vi "Test Arduino-Adafruit stepper API.vi"() -> ()   [LabVIEW 2020]
doc: "Arduino-Adafruit stepper API Tester."
uses:
  Arduino stepper library/Public/Controls/Com Port Options.ctl
  Arduino stepper library/Public/Controls/Motor initialization parameters--cluster.ctl
  Arduino stepper library/Public/Controls/Motor direction.ctl
  Arduino stepper library/Public/Controls/Move motor parameters--cluster.ctl
  Arduino stepper library/Public/Controls/Step style.ctl
  <vilib>/Utility/error.llb/DialogType.ctl
  Arduino-Adafruit stepper.lvlib
  Arduino stepper library/Control de MaP.lvlib
panel:
  in  "Stop movement":bool
  in  "Timeout":i32=50
  in  "Move parameters":T1={"Action"=1, "Direction motor 1"=1, "Direction motor 2"=1, "Steps motor 1"=200, "Steps motor 2"=200, "Step style motor 1"=1, "Step style motor 2"=1} {"Step style motor 2" items=["", "Single", "Double", "Interleave", "Microstep"]; "Step style motor 1" items=["", "Single", "Double", "Interleave", "Microstep"]; "Direction motor 2" items=["", "Forward", "Backward"]; "Direction motor 1" items=["", "Forward", "Backward"]; "Action" items=["", "Initialize", "Move"]}
  in  "Begin movement":bool
  in  "Home direction (M2)":T2=1 items=["", "Forward", "Backward"]
  in  "Home direction (M1)":T2=1 items=["", "Forward", "Backward"]
  in  "Home motors":bool
  out "Motors ready?":bool
  in  "Comando":T4={"Action"=0, "Steps per rev motor 1"=200, "Steps per rev motor 2"=200, "RPM motor 1"=400, "RPM motor 2"=400} {"Action" items=["Initialize", "Move"]}
  in  "Init motors":bool
  out "Connected?":bool
  in  "Disconnect":bool
  in  "COM options":T5={"baud rate"=115200, "data bits"=8, "parity"=enum."None"} {"data bits" min=5 max=8 step=1}
  in  "VISA resource name":refnum<visa-resource-name>
  in  "Connect":bool
  out "last error":errorcluster
  in  "Show Diagram on Init":bool
  in  "Run as Singleton?":bool
  in  "Show Block Diagram":bool
  in  "Refresh Modules":bool
  out "Active Modules":string[](array[string])
  in  "Stop Module":bool
  in  "Select Module":i32(ring)=-1 caption="Select Module\nTo send Request to" items=["All"=-1]
  in  "Run New Module":bool
  in  "Hide Module Panel":bool
  in  "Show Module Panel":bool
  out "Status":string
  # "This VI tests the API for the Module."
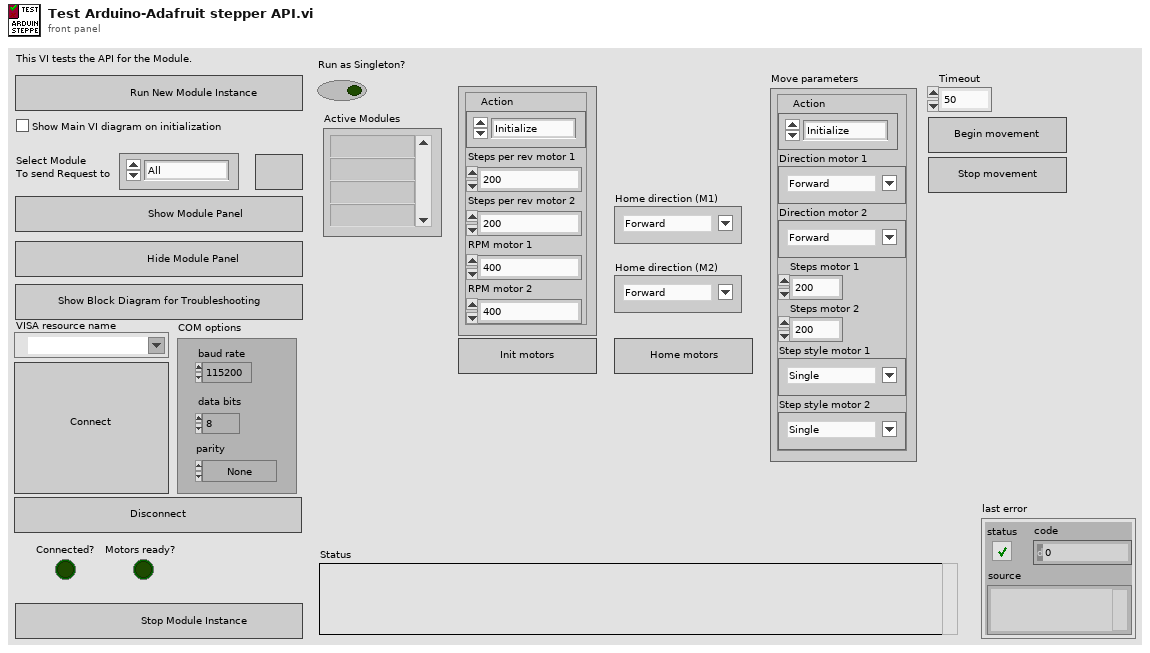
[diagram p1: front panel]
types:
  T1 = typedef "Control de MaP.lvlib/Move motor parameters--cluster.ctl" = cluster{"Action":u8, "Direction motor 1":T2, "Direction motor 2":T2, "Steps motor 1":u16, "Steps motor 2":u16, "Step style motor 1":T3, "Step style motor 2":T3}
  T2 = typedef "Control de MaP.lvlib/Motor direction.ctl" = u8
  T3 = typedef "Control de MaP.lvlib/Step style.ctl" = u8
  T4 = typedef "Control de MaP.lvlib/Motor initialization parameters--cluster.ctl" = cluster{"Action":u8, "Steps per rev motor 1":u8, "Steps per rev motor 2":u8, "RPM motor 1":u16, "RPM motor 2":u16}
  T5 = typedef "Control de MaP.lvlib/Com Port Options.ctl" = cluster{"baud rate":u32, "data bits":u16, "parity":enum16{"None", "Odd", "Even", "Mark", "Space"}}
  T6 = typedef "Arduino-Adafruit stepper.lvlib/Broadcast Events--cluster.ctl" = cluster{"Module Did Init":refnum<user-event>, "Status Updated":refnum<user-event>, "Error Reported":refnum<user-event>, "Module Did Stop":refnum<user-event>, "Update Module Execution Status":refnum<user-event>, "Connection successful":refnum<user-event>, "Connection failed":refnum<user-event>, "Device disconnected":refnum<user-event>, "Motors ready":refnum<user-event>, "System busy":refnum<user-event>}
  T7 = typedef "DialogType.ctl" = u16
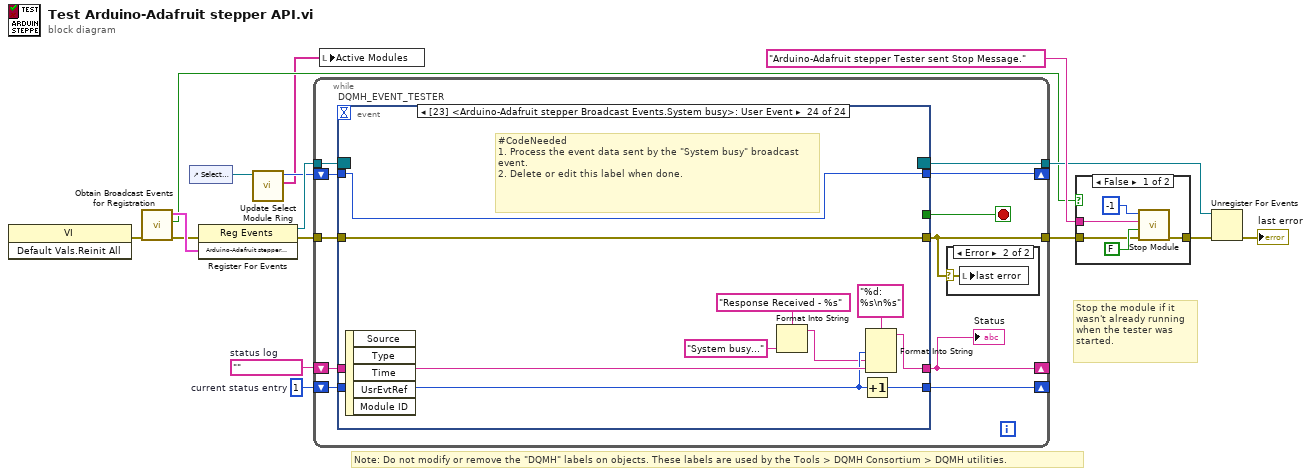
[diagram p0: block diagram]
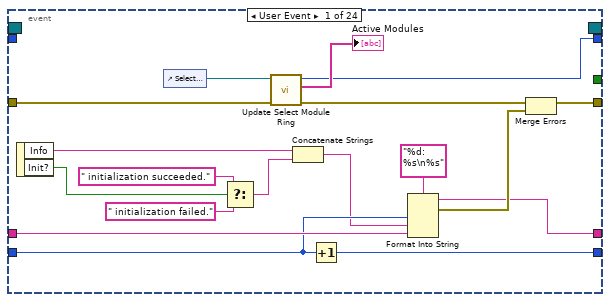
[diagram p4: hidden frame]
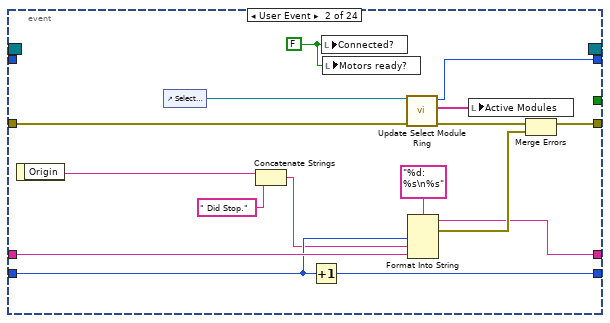
[diagram p5: hidden frame]
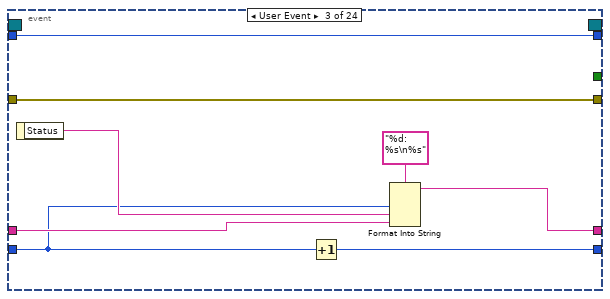
[diagram p6: hidden frame]
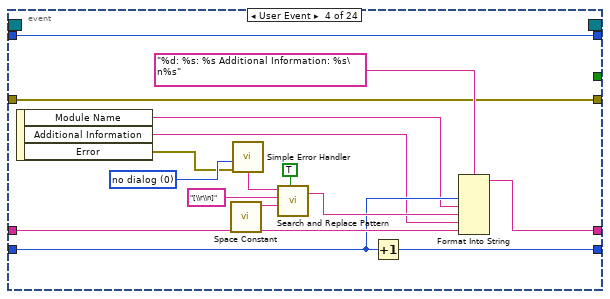
[diagram p7: hidden frame]
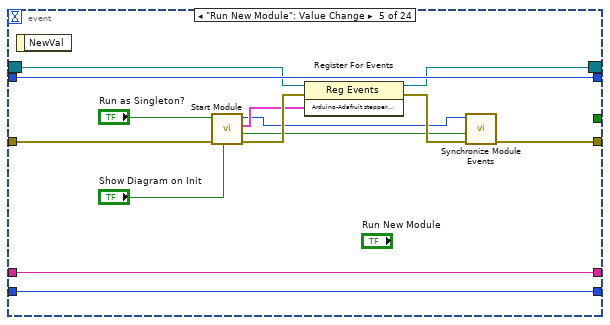
[diagram p8: hidden frame]
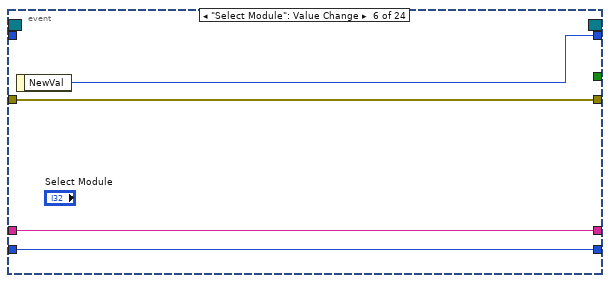
[diagram p9: hidden frame]
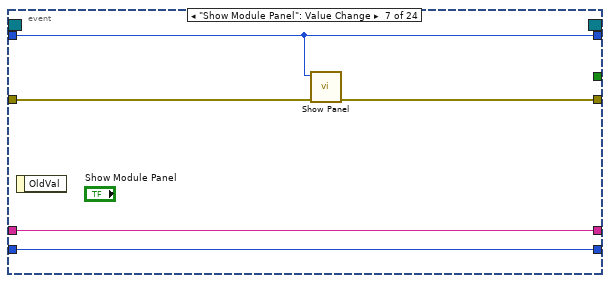
[diagram p10: hidden frame]
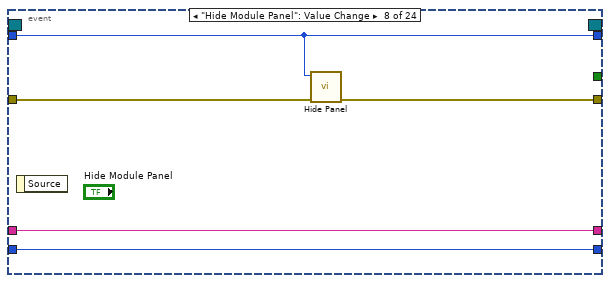
[diagram p11: hidden frame]
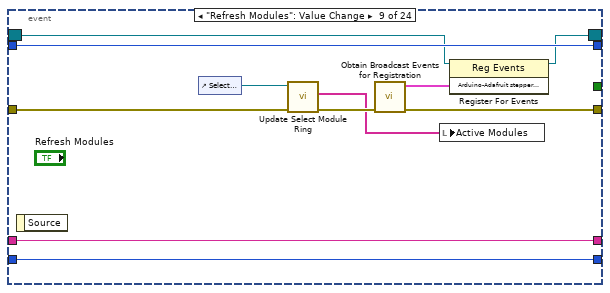
[diagram p12: hidden frame]
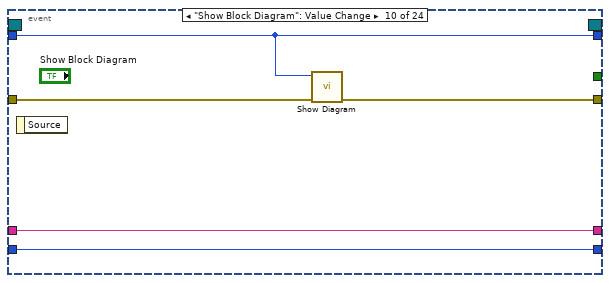
[diagram p13: hidden frame]
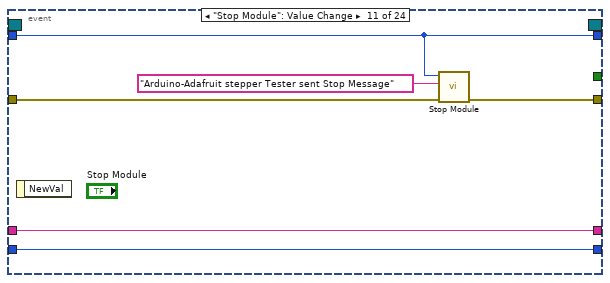
[diagram p14: hidden frame]
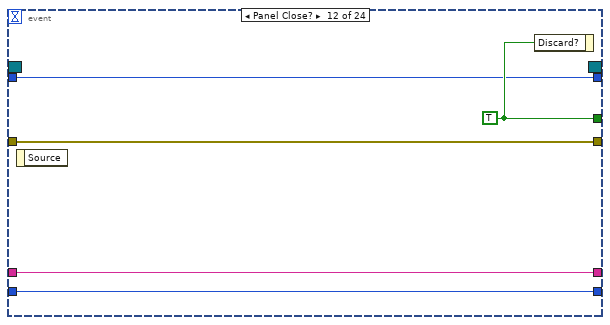
[diagram p15: hidden frame]
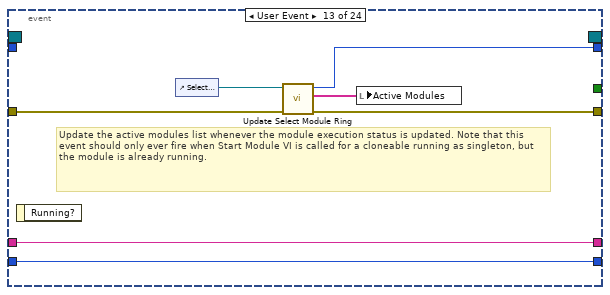
[diagram p16: hidden frame]
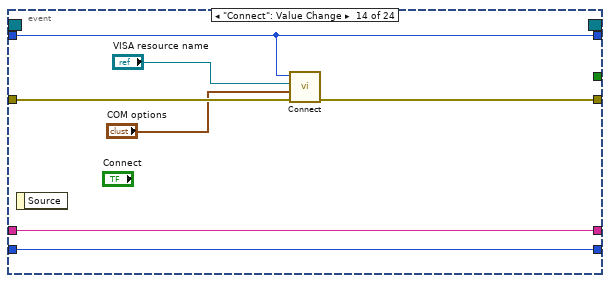
[diagram p17: hidden frame]
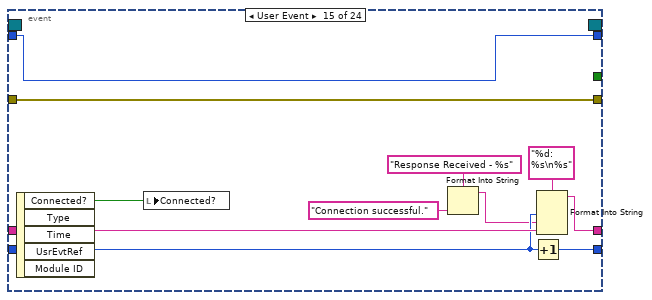
[diagram p18: hidden frame]
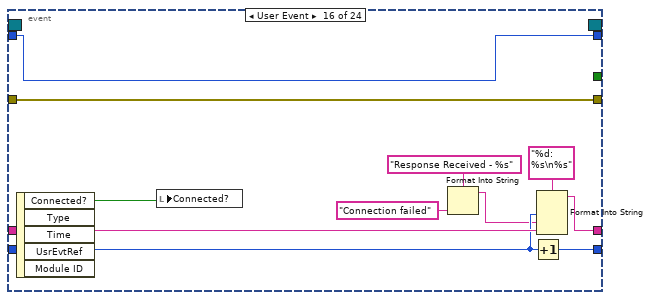
[diagram p19: hidden frame]
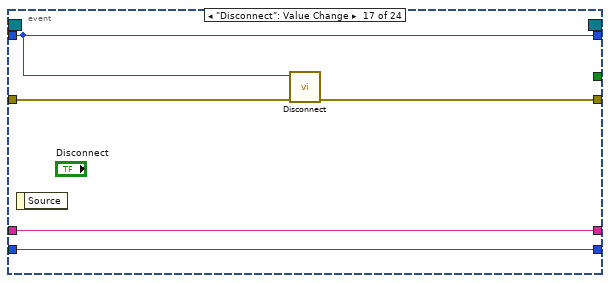
[diagram p20: hidden frame]
diagram:
  w13 = 1  # current status entry
  w14 = ""  # status log
  # "Stop the module if it wasn't already running when the tester was started."
  # "Note: Do not modify or remove the \"DQMH\" labels on objects. These labels are used by the Tools > DQMH Consortium > DQMH utilities."
  n1 = invoke class="VI" method="Default Vals.Reinit All"() -> (error out=w8:errorcluster)  [unwired: 3 in, 2 out]
  n2 = call "Obtain Broadcast Events for Registration.vi"("error in"=w8) -> ("error out"=w7:errorcluster, "Already running?"=w6:bool, "Arduino-Adafruit stepper Broadcast Events"=w12:T6)  [unwired: 8 in]
  n3 = control-ref of="Select Module"() -> (w3:refnum<vi>)
  n4 = register-events(error in=w7, w12) -> (reference out=w16:refnum<event-registration>, error out=w11:errorcluster)  [unwired: 1 in]
  n5 = call "Update Select Module Ring.vi"("Select Module Ring Ref"=w3) -> ("Active Modules (Array)"=w1:string[], "New Module Ring Value"=w2:i32)  [unwired: 8 in, 1 out]
  n6 = while {
    tunnel: w16 -> [w27]
    tunnel: [w18] -> w5
    tunnel: w11 -> [w26]
    shift-right: [w22] -> _
    shift-left: w14 -> [w24]
    shift-right: [w23] -> _
    shift-left: w13 -> [w25]
    shift-right: [w20] -> _
    shift-left: w2 -> [w21]
    tunnel: [w19] -> w9
    stop <- w17 stop-if-true
    n7 = event "DQMH_EVENT_TESTER" shown="[23] <Arduino-Adafruit stepper Broadcast Events.System busy>: User Event" {
      selector: w27 -> [_ _ _ _ w94 _ _ _ w120 _ _ _ _ _ _ _ _ _ _ _ _ _ _ _]
      dyn-events: [_ _ _ _ w93 _ _ _ w119 _ _ _ _ _ _ _ _ _ _ _ _ _ _ _] -> w19
      timeout: _ -> [_ _ _ _ _ _ _ _ _ _ _ _ _ _ _ _ _ _ _ _ _ _ _ _]
      tunnel: [_ _ _ _ _ _ _ _ _ _ _ w141 _ _ _ _ _ _ _ _ _ _ _ _] -> w17
      tunnel: [w36 w54 w70 w74 w92 w104 w108 w113 w116 w127 w132 w140 w144 w151 w166 w177 w178 w193 w195 w210 w213 w220 w225 w239] -> w18
      tunnel: w26 -> [w38 w56 w70 w74 w95 w104 w109 w114 w121 w130 w133 w140 w145 w155 w166 w177 w182 w193 w199 w210 w217 w224 w229 w239]
      tunnel: w25 -> [w43 w59 w63 w77 w97 w102 w106 w111 w124 w128 w135 w138 w147 w153 w162 w173 w180 w189 w197 w206 w215 w222 w227 w235]
      tunnel: w24 -> [w44 w60 w66 w78 w98 w103 w107 w112 w125 w129 w136 w139 w148 w154 w164 w175 w181 w191 w198 w208 w216 w223 w228 w237]
      tunnel: [w41 w57 w67 w76 w98 w103 w107 w112 w125 w129 w136 w139 w148 w154 w163 w174 w181 w190 w198 w207 w216 w223 w228 w236] -> w22
      tunnel: [w42 w58 w69 w75 w97 w102 w106 w111 w124 w128 w135 w138 w147 w153 w161 w172 w180 w188 w197 w205 w215 w222 w227 w234] -> w23
      tunnel: w21 -> [_ _ w64 w86 w96 _ w105 w110 w123 w126 w134 w137 _ w152 w165 w176 w179 w192 w196 w209 w214 w221 w226 w238]
      tunnel: [w33 w51 w64 w86 w96 w101 w105 w110 w123 w126 w134 w137 w143 w152 w165 w176 w179 w192 w196 w209 w214 w221 w226 w238] -> w20
      event User Event {
        n8 = event-data() -> ("Info"=w40:string, "Init?"=w30:bool)  [unwired: 1 in]
        n9 = control-ref of="Select Module"() -> (w35:refnum<vi>)
        n10 = Select(t=" initialization succeeded.", s=w30, f=" initialization failed.") -> (s? t:f=w29:string)
        n11 = call "Update Select Module Ring.vi"("error in"=w38, "Select Module Ring Ref"=w35) -> ("error out"=w37:errorcluster, "Active Modules (Array)"=→"Active Modules":string[], "New Module Ring Value"=w33:i32)  [unwired: 7 in]
        n12 = Concatenate Strings(w40, w29) -> (w39:string)
        n13 = Increment(x=w43) -> (x+1=w42:i32)
        n14 = Format Into String(format string="%d: %s\n%s", w43, w39, w44) -> (resulting string=w41:string, error out=w46:errorcluster)  [unwired: 2 in]
        n15 = Merge Errors(w37, w46) -> (w36:errorcluster)
      }
      event User Event {
        w47 = FALSE ("Connected?")
        n16 = event-data() -> ("Origin"=w49:string)  [unwired: 1 in]
        n17 = control-ref of="Select Module"() -> (w53:refnum<vi>)
        n18 = Concatenate Strings(w49, " Did Stop.") -> (w48:string)
        n19 = Increment(x=w59) -> (x+1=w58:i32)
        n20 = local write "Connected?"(w47) -> ()
        n21 = local write "Motors ready?"(w47) -> ()
        n22 = call "Update Select Module Ring.vi"("error in"=w56, "Select Module Ring Ref"=w53) -> ("error out"=w55:errorcluster, "Active Modules (Array)"=w52:string[], "New Module Ring Value"=w51:i32)  [unwired: 7 in]
        n23 = Format Into String(format string="%d: %s\n%s", w59, w48, w60) -> (resulting string=w57:string, error out=w62:errorcluster)  [unwired: 2 in]
        n24 = local write "Active Modules"(w52) -> ()
        n25 = Merge Errors(w55, w62) -> (w54:errorcluster)
      }
      event User Event {
        n26 = event-data() -> ("Status"=w65:string)  [unwired: 1 in]
        n27 = Increment(x=w63) -> (x+1=w69:i32)
        n28 = Format Into String(format string="%d: %s\n%s", w63, w65, w66) -> (resulting string=w67:string)  [unwired: 2 in, 1 out]
      }
      event User Event {
        w79 = T7 0 items=["no dialog", "OK message", "continue or stop message", "OK message + warnings", "continue/stop + warnings"] ("type of dialog (OK msg:1)")
        n29 = event-data() -> ("Module Name"=w73:string, "Additional Information"=w72:string, "Error"=w71:errorcluster)  [unwired: 1 in]
        n30 = call <vilib>:"Space Constant.vi"() -> ("String"=w83:string)
        n31 = call <vilib>:"Simple Error Handler.vi"("type of dialog (OK msg:1)"=w79, "error in (no error)"=w71) -> ("message"=w80:string)  [unwired: 3 in, 4 out]
        n32 = call <vilib>:"Search and Replace Pattern.vi"("string"=w80, "regular expression (\"\")"="[\\r\\n]" ("regular expression (\"\")"), "replace string (\"\")"=w83, "replace all? (F)"=TRUE ("replace all CR/LF with spaces")) -> ("result string"=w81:string)  [unwired: 1 in, 1 out]
        n33 = Increment(x=w77) -> (x+1=w75:i32)
        n34 = Format Into String(format string="%d: %s: %s Additional Information: %s\n%s", w77, w73, w81, w72, w78) -> (resulting string=w76:string)  [unwired: 2 in, 1 out]
      }
      event "Run New Module": Value Change {
        n35 = event-data() -> ()  [unwired: 1 in, 1 out]
        n36 = call "Start Module.vi"("Show Main VI Diagram on Init (F)"="Show Diagram on Init", "error in"=w95, "Run as Singleton? (F)"="Run as Singleton?") -> ("error out"=w99:errorcluster, "Wait for Event Sync?"=w91:bool, "Arduino-Adafruit stepper Broadcast Events"=w90:T6, "Module ID"=w87:i32)  [unwired: 5 in]
        n37 = register-events(reference=w94, error in=w99, w90) -> (reference out=w93:refnum<event-registration>, error out=w100:errorcluster)
        n38 = call "Synchronize Module Events.vi"("error in"=w100, "Wait for Event Sync?"=w91, "Module ID in"=w87) -> ("error out"=w92:errorcluster)  [unwired: 7 in, 1 out]
      }
      event "Select Module": Value Change {
        n39 = event-data() -> ("NewVal"=w101:i32)  [unwired: 1 in]
      }
      event "Show Module Panel": Value Change {
        n40 = event-data() -> ()  [unwired: 1 in, 1 out]
        n41 = call "Show Panel.vi"("error in"=w109, "Module ID"=w105) -> ("error out"=w108:errorcluster)  [unwired: 9 in]
      }
      event "Hide Module Panel": Value Change {
        n42 = event-data() -> ()  [unwired: 1 in, 1 out]
        n43 = call "Hide Panel.vi"("error in"=w114, "Module ID"=w110) -> ("error out"=w113:errorcluster)  [unwired: 9 in]
      }
      event "Refresh Modules": Value Change {
        n44 = event-data() -> ()  [unwired: 1 in, 1 out]
        n45 = control-ref of="Select Module"() -> (w122:refnum<vi>)
        n46 = call "Update Select Module Ring.vi"("error in"=w121, "Select Module Ring Ref"=w122) -> ("error out"=w117:errorcluster, "Active Modules (Array)"=w115:string[])  [unwired: 7 in, 1 out]
        n47 = call "Obtain Broadcast Events for Registration.vi"("error in"=w117) -> ("error out"=w116:errorcluster, "Arduino-Adafruit stepper Broadcast Events"=w118:T6)  [unwired: 8 in, 1 out]
        n48 = local write "Active Modules"(w115) -> ()
        n49 = register-events(reference=w120, w118) -> (reference out=w119:refnum<event-registration>)  [unwired: 1 in, 1 out]
      }
      event "Show Block Diagram": Value Change {
        n50 = event-data() -> ()  [unwired: 1 in, 1 out]
        n51 = call "Show Diagram.vi"("error in"=w130, "Module ID"=w126) -> ("error out"=w127:errorcluster)  [unwired: 9 in]
      }
      event "Stop Module": Value Change {
        n52 = event-data() -> ()  [unwired: 1 in, 1 out]
        n53 = call "Stop Module.vi"("error in"=w133, "Origin"="Arduino-Adafruit stepper Tester sent Stop Message", "Module ID"=w134) -> ("error out"=w132:errorcluster)  [unwired: 8 in]
      }
      event Panel Close? {
        w141 = TRUE ("Discard?")
        n54 = event-data() -> ()  [unwired: 1 in, 1 out]
        n55 = event-data("Discard?"=w141) -> ()  [unwired: 1 in, 1 out]
      }
      event User Event {
        # "Update the active modules list whenever the module execution status is updated. Note that this event should only ever fire when Start Module VI is called for a cloneable running as singleton, but the module is already running."
        n56 = event-data() -> ()  [unwired: 1 in, 1 out]
        n57 = control-ref of="Select Module"() -> (w146:refnum<vi>)
        n58 = call "Update Select Module Ring.vi"("error in"=w145, "Select Module Ring Ref"=w146) -> ("error out"=w144:errorcluster, "Active Modules (Array)"=w142:string[], "New Module Ring Value"=w143:i32)  [unwired: 7 in]
        n59 = local write "Active Modules"(w142) -> ()
      }
      event "Connect": Value Change {
        n60 = event-data() -> ()  [unwired: 1 in, 1 out]
        n61 = call "Connect.vi"("error in"=w155, "COM options"="COM options", "VISA resource name"="VISA resource name", "Module ID"=w152) -> ("error out"=w151:errorcluster)  [unwired: 7 in]
      }
      event User Event {
        n62 = event-data() -> ("Connected?"=w156:bool)  [unwired: 1 in, 4 out]
        n63 = local write "Connected?"(w156) -> ()
        n64 = Format Into String(format string="Response Received - %s", "Connection successful." ("input 1")) -> (resulting string=w158:string)  [unwired: 2 in, 1 out]
        n65 = Increment(x=w162) -> (x+1=w161:i32)
        n66 = Format Into String(format string="%d: %s\n%s", w162, w158, w164) -> (resulting string=w163:string)  [unwired: 2 in, 1 out]
      }
      event User Event {
        n67 = event-data() -> ("Connected?"=w167:bool)  [unwired: 1 in, 4 out]
        n68 = local write "Connected?"(w167) -> ()
        n69 = Format Into String(format string="Response Received - %s", "Connection failed" ("input 1")) -> (resulting string=w169:string)  [unwired: 2 in, 1 out]
        n70 = Increment(x=w173) -> (x+1=w172:i32)
        n71 = Format Into String(format string="%d: %s\n%s", w173, w169, w175) -> (resulting string=w174:string)  [unwired: 2 in, 1 out]
      }
      event "Disconnect": Value Change {
        n72 = event-data() -> ()  [unwired: 1 in, 1 out]
        n73 = call "Disconnect.vi"("error in"=w182, "Module ID"=w179) -> ("error out"=w178:errorcluster)  [unwired: 9 in]
      }
      event User Event {
        n74 = event-data() -> ("Connected?"=w183:bool)  [unwired: 1 in, 4 out]
        "Connected?" <- w183
        n75 = local write "Motors ready?"(w183) -> ()
        n76 = Format Into String(format string="Response Received - %s", "Device disconnected." ("input 1")) -> (resulting string=w185:string)  [unwired: 2 in, 1 out]
        n77 = Increment(x=w189) -> (x+1=w188:i32)
        n78 = Format Into String(format string="%d: %s\n%s", w189, w185, w191) -> (resulting string=w190:string)  [unwired: 2 in, 1 out]
      }
      event "Init motors": Value Change {
        n79 = event-data() -> ()  [unwired: 1 in, 1 out]
        n80 = call "Init motors.vi"("error in"=w199, "Comando"="Comando", "Module ID"=w196) -> ("error out"=w195:errorcluster)  [unwired: 8 in]
      }
      event User Event {
        n81 = event-data() -> ("Motors ready?"=→"Motors ready?":bool)  [unwired: 1 in, 4 out]
        n82 = Format Into String(format string="Response Received - %s", "Motors ready and standing by." ("input 1")) -> (resulting string=w202:string)  [unwired: 2 in, 1 out]
        n83 = Increment(x=w206) -> (x+1=w205:i32)
        n84 = Format Into String(format string="%d: %s\n%s", w206, w202, w208) -> (resulting string=w207:string)  [unwired: 2 in, 1 out]
      }
      event "Home motors": Value Change {
        n85 = event-data() -> ()  [unwired: 1 in, 1 out]
        n86 = call "Home motors.vi"("error in"=w217, "Home direction (M2)"="Home direction (M2)", "Home direction (M1)"="Home direction (M1)", "Module ID"=w214) -> ("error out"=w213:errorcluster)  [unwired: 7 in]
      }
      event "Begin movement": Value Change {
        n87 = event-data() -> ()  [unwired: 1 in, 1 out]
        n88 = call "Begin movement.vi"("error in"=w224, "Timeout"="Timeout", "Move parameters"="Move parameters", "Module ID"=w221) -> ("error out"=w220:errorcluster)  [unwired: 7 in]
      }
      event "Stop movement": Value Change {
        n89 = event-data() -> ()  [unwired: 1 in, 1 out]
        n90 = call "Stop movement.vi"("error in"=w229, "Module ID"=w226) -> ("error out"=w225:errorcluster)  [unwired: 9 in]
      }
      event User Event {
        # "#CodeNeeded\n1. Process the event data sent by the \"System busy\" broadcast event.\n2. Delete or edit this label when done."
        n91 = event-data() -> ()  [unwired: 1 in, 5 out]
        n92 = Format Into String(format string="Response Received - %s", "System busy..." ("input 1")) -> (resulting string=w231:string)  [unwired: 2 in, 1 out]
        n93 = Increment(x=w235) -> (x+1=w234:i32)
        n94 = Format Into String(format string="%d: %s\n%s", w235, w231, w237) -> (resulting string=w236:string)  [unwired: 2 in, 1 out]
      }
    }
    "Status" <- w22
    n95 = case shown="Error" w18 {
      selector: w18 -> [_ w28]
      frame No Error {
      }
      frame Error {
        n96 = local write "last error"(w28) -> ()
      }
    }
  }
  n97 = local write "Active Modules"(w1) -> ()
  n98 = case shown="False" w6 {
    tunnel: [w244 w245] -> w15
    tunnel: "Arduino-Adafruit stepper Tester sent Stop Message." ("Origin") -> [w243 _]
    tunnel: w5 -> [w240 w245]
    frame False {
      n99 = call "Stop Module.vi"("error in"=w240, "Wait for Module to stop? (F)"=FALSE ("Wait for Module to stop?"), "Origin"=w243, "Module ID"=-1 ("Stop all")) -> ("error out"=w244:errorcluster)  [unwired: 7 in]
    }
    frame True {
    }
  }
  n100 = Unregister For Events(event registration refnum=w9, error in=w15) -> (error out=→"last error":errorcluster)
